vi "solar_misc Netstat Query.vi"(8 "error in (no error)":errorcluster) -> (0 "error out":errorcluster, 3 "netstat":T1(array[cluster]))   [LabVIEW 2018]
doc: "This VI queries the network stack and list the state of each active network connection.\n\nCreated By: Ryan Pacini"
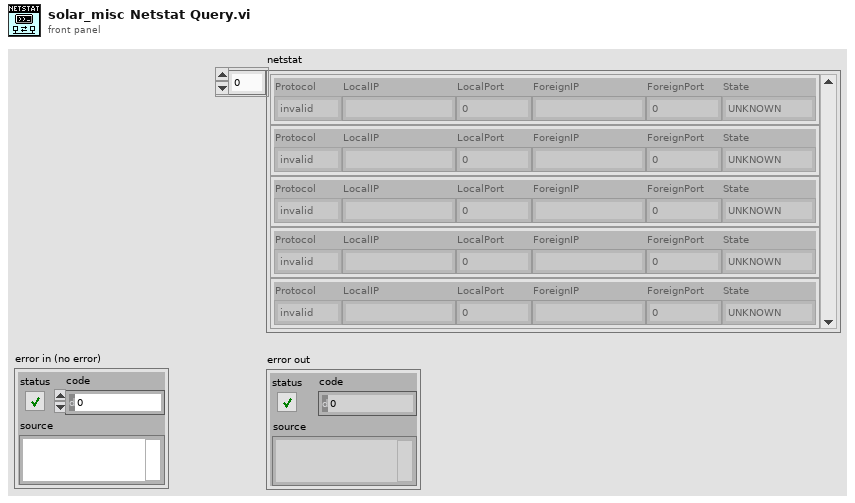
[diagram p1: front panel]
types:
  T1 = cluster{"Protocol":enum16{"invalid", "tcp", "udp", "icmp", "ip", "tcpv6", "udpv6", "icmpv6", "ipv6"}, "LocalIP":string, "LocalPort":u16, "ForeignIP":string, "ForeignPort":u16, "State":enum8{"UNKNOWN", "LISTEN", "ESTABLISHED", "SYN_SENT", "SYN_RECV", "LAST_ACK", "CLOSE_WAIT", "TIME_WAIT", "CLOSED", "CLOSING", "FIN_WAIT1", "FIN_WAIT2"}}[]
  T2 = enum16{"invalid", "tcp", "udp", "icmp", "ip", "tcpv6", "udpv6", "icmpv6", "ipv6"}
  T3 = cluster{"Protocol":enum16{"invalid", "tcp", "udp", "icmp", "ip", "tcpv6", "udpv6", "icmpv6", "ipv6"}, "LocalIP":string, "LocalPort":u16, "ForeignIP":string, "ForeignPort":u16, "State":enum8{"UNKNOWN", "LISTEN", "ESTABLISHED", "SYN_SENT", "SYN_RECV", "LAST_ACK", "CLOSE_WAIT", "TIME_WAIT", "CLOSED", "CLOSING", "FIN_WAIT1", "FIN_WAIT2"}}
  T4 = enum8{"UNKNOWN", "LISTEN", "ESTABLISHED", "SYN_SENT", "SYN_RECV", "LAST_ACK", "CLOSE_WAIT", "TIME_WAIT", "CLOSED", "CLOSING", "FIN_WAIT1", "FIN_WAIT2"}
  T5 = cluster{"LocalPort":u16, "netstat":cluster{"Protocol":enum16{"invalid", "tcp", "udp", "icmp", "ip", "tcpv6", "udpv6", "icmpv6", "ipv6"}, "LocalIP":string, "LocalPort":u16, "ForeignIP":string, "ForeignPort":u16, "State":enum8{"UNKNOWN", "LISTEN", "ESTABLISHED", "SYN_SENT", "SYN_RECV", "LAST_ACK", "CLOSE_WAIT", "TIME_WAIT", "CLOSED", "CLOSING", "FIN_WAIT1", "FIN_WAIT2"}}}
  T6 = cluster{"LocalPort":u16, "netstat":cluster{"Protocol":enum16{"invalid", "tcp", "udp", "icmp", "ip", "tcpv6", "udpv6", "icmpv6", "ipv6"}, "LocalIP":string, "LocalPort":u16, "ForeignIP":string, "ForeignPort":u16, "State":enum8{"UNKNOWN", "LISTEN", "ESTABLISHED", "SYN_SENT", "SYN_RECV", "LAST_ACK", "CLOSE_WAIT", "TIME_WAIT", "CLOSED", "CLOSING", "FIN_WAIT1", "FIN_WAIT2"}}}[]
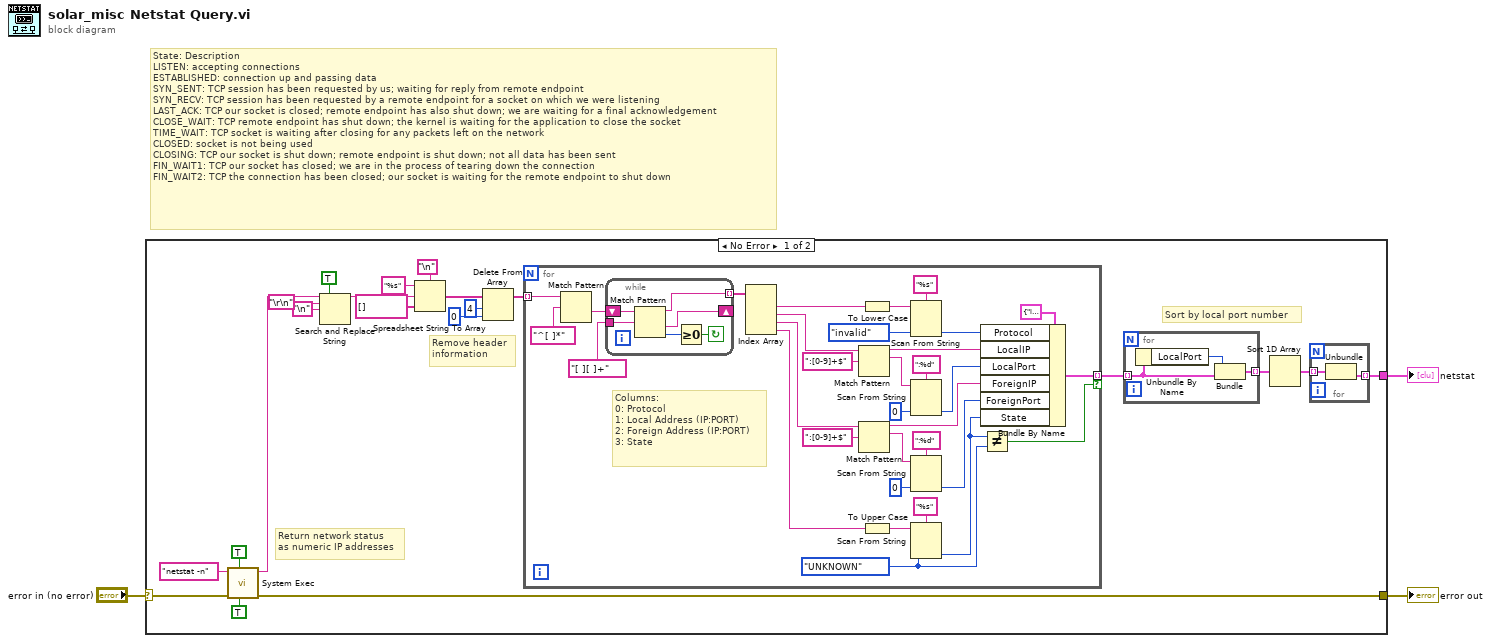
[diagram p0: block diagram]
diagram:
  # "State: Description\nLISTEN: accepting connections\nESTABLISHED: connection up and passing data\nSYN_SENT: TCP session has been requested by us; waiting for reply from remote endpoint\nSYN_RECV: TCP session has been requested by a remote endpoint for a socket on which we were listening\nLAST_ACK: TCP our socket is closed; remote endpoint has also shut down; we are waiting for a final acknowledgement\nCLOSE_WAIT: TCP remote endpoint has shut down; the kernel is waiting for the application to close the socket\nTIME_WAIT: TCP socket is waiting after closing for any packets left on the network\nCLOSED: socket is not being used\nCLOSING: TCP our socket is shut down; remote endpoint is shut down; not all data has been sent\nFIN_WAIT1: TCP our socket has closed; we are in the process of tearing down the connection\nFIN_WAIT2: TCP the connection has been closed; our socket is waiting for the remote endpoint to shut down"
  n1 = case shown="No Error" "error in (no error)" {
    selector: "error in (no error)" -> [w22 w68]
    tunnel: [w21 w68] -> w2
    tunnel: [w4 _] -> w1
    frame No Error {
      # "Sort by local port number"
      # "Return network status\nas numeric IP addresses"
      # "Remove header\ninformation"
      n2 = call <vilib>:"System Exec.vi"("run minimized? (F)"=TRUE, "wait until completion? (T)"=TRUE, "error in (no error)"=w22, "command line"="netstat -n") -> ("error out"=w21:errorcluster, "standard output"=w19:string)  [unwired: 4 in, 2 out]
      n3 = Search and Replace String(replace all?=TRUE ("replace all? (F)"), input string=w19, search string="\r\n" ("End of Line Constant"), replace string="\n" ("Line Feed Constant")) -> (result string=w15:string)  [unwired: 4 in, 3 out]
      n4 = Spreadsheet String To Array(delimiter (Tab)="\n", format string="%s", spreadsheet string=w15, array type (2D Dbl)=string[] []) -> (array=w11:string[])
      n5 = Delete From Array(array=w11, length=4, index=0) -> (array with subset deleted=w10:string[])  [unwired: 1 out]
      n6 = for {
        tunnel: w10 -> [w54] mode=indexing
        tunnel: [w55] -> w5 mode=indexing if=w32
        w30 = T4."UNKNOWN" ("State")
        # "Columns:\n0: Protocol\n1: Local Address (IP:PORT)\n2: Foreign Address (IP:PORT)\n3: State"
        n7 = Match Pattern(string=w54, regular expression="^[ ]*") -> (after substring=w53:string)  [unwired: 1 in, 3 out]
        n8 = while {
          shift-right: [w65] -> _
          shift-left: w53 -> [w66]
          tunnel: [w64] -> w60 mode=indexing
          tunnel: "[ ][ ]+" ("regular expression") -> [w62]
          stop <- w63 continue-if-true
          n9 = Match Pattern(string=w66, regular expression=w62) -> (before substring=w64:string, after substring=w65:string, offset past match=w67:i32)  [unwired: 1 in, 1 out]
          n10 = Greater Or Equal To 0?(x=w67) -> (x >= 0?=w63:bool)
        }
        n11 = Index Array(array=w60) -> (element #1=w58:string, element #2=w51:string, element #3=w42:string, element #4=w38:string)  [unwired: 4 in]
        n12 = Match Pattern(string=w51, regular expression=":[0-9]+$") -> (before substring=w49:string, match substring=w35:string)  [unwired: 1 in, 2 out]
        n13 = Match Pattern(string=w42, regular expression=":[0-9]+$") -> (before substring=w41:string, match substring=w36:string)  [unwired: 1 in, 2 out]
        n14 = To Lower Case(string=w58) -> (all lower case string=w56:string)
        n15 = To Upper Case(1:w38) -> (0:w37:string)
        n16 = Scan From String(format string="%s", input string=w56, default 1=T2."invalid" ("Protocol")) -> (output 1=w34:T2)  [unwired: 2 in, 3 out]
        n17 = Scan From String(format string=":%d", input string=w35, default 1=u16 0 ("default value 1")) -> (output 1=w46:u16)  [unwired: 2 in, 3 out]
        n18 = Scan From String(format string=":%d", input string=w36, default 1=u16 0 ("default value 1")) -> (output 1=w40:u16)  [unwired: 2 in, 3 out]
        n19 = Scan From String(format string="%s", input string=w37, default 1=w30) -> (output 1=w31:T4)  [unwired: 2 in, 3 out]
        n20 = Bundle By Name(cluster=T3 {"Protocol"=enum."invalid", "LocalIP"="", "LocalPort"=0, "ForeignIP"="", "ForeignPort"=0, "State"=enum."UNKNOWN"} ("netstat"), "Protocol"=w34, "LocalIP"=w49, "LocalPort"=w46, "ForeignIP"=w41, "ForeignPort"=w40, "State"=w31) -> (w55:T3)
        n21 = Not Equal?(x=w31, y=w30) -> (x != y?=w32:bool)
      }
      n22 = for {
        tunnel: w5 -> [w28] mode=indexing
        tunnel: [w27] -> w7 mode=indexing
        n23 = Unbundle By Name(w28) -> ("LocalPort"=w29:u16)
        n24 = Bundle("LocalPort"=w29, "netstat"=w28) -> (w27:T5)  [unwired: 1 in]
      }
      n25 = Sort 1D Array(array=w7) -> (sorted array=w6:T6)
      n26 = for {
        tunnel: w6 -> [w26] mode=indexing
        tunnel: [w25] -> w4 mode=indexing
        n27 = Unbundle(w26) -> ("netstat"=w25:T3)  [unwired: 1 out]
      }
    }
    frame Error {
    }
  }
  "error out" <- w2
  "netstat" <- w1
